vi "reading_csv.vi"() -> ()   [LabVIEW 2024]
uses:
  <vilib>/Utility/file.llb/Read Delimited Spreadsheet (string).vi
panel:
  out "Array":T1(array[cluster])
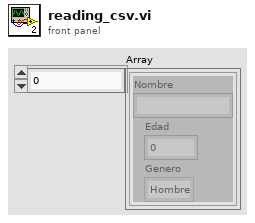
[diagram p1: front panel]
types:
  T1 = cluster{"Nombre":string, "Edad":i32, "Genero":enum16{"Mujer", "Hombre"}}[]
  T2 = cluster{"Nombre":string, "Edad":i32, "Genero":enum16{"Mujer", "Hombre"}}
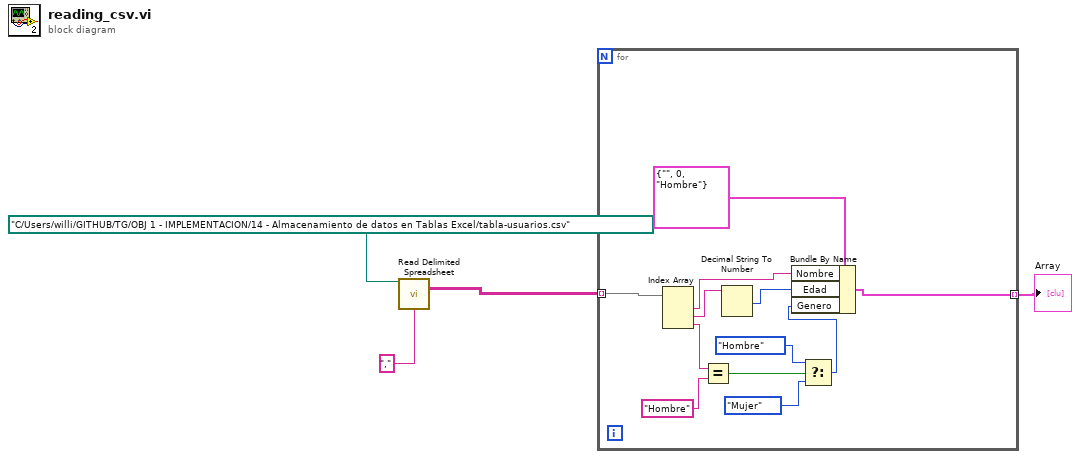
[diagram p0: block diagram]
diagram:
  n1 = call-poly <vilib>:"Read Delimited Spreadsheet.vi"("file path (dialog if empty)"=path "C:/Users/willi/GITHUB/TG/OBJ 1 - IMPLEMENTACION/14 - Almacenamiento de datos en Tablas Excel/tabla-usuarios.csv", "delimiter (\\t)"="," ("delimiter (\\t)")) -> ("all rows"=w2:string[][])  [unwired: 8 in, 5 out]
  n2 = for {
    tunnel: w2 -> [w16] mode=indexing
    tunnel: [w5] -> w1 mode=indexing
    n3 = Index Array(array=w16) -> (element #1=w14:string, element #2=w13:string, element #3=w10:string)  [unwired: 3 in]
    n4 = Equal?(x=w10, y="Hombre") -> (x = y?=w9:bool)
    n5 = Decimal String To Number(string=w13) -> (number=w12:i32)  [unwired: 2 in, 1 out]
    n6 = Select(t=enum16{"Mujer", "Hombre"}."Hombre" ("Genero"), s=w9, f=enum16{"Mujer", "Hombre"}."Mujer" ("Genero")) -> (s? t:f=w6:enum16{"Mujer", "Hombre"})
    n7 = Bundle By Name(cluster=T2 {"Nombre"="", "Edad"=0, "Genero"=enum."Hombre"} ("Detalles de la Persona"), "Nombre"=w14, "Edad"=w12, "Genero"=w6) -> (w5:T2)
  }
  "Array" <- w1
